vi "test Check If Custom Device is Enabled.vi"(8 "error in":errorcluster, 11 "TestCase in":refnum<class "Scripting.lvclass">) -> (0 "error out":errorcluster)   [LabVIEW 2020, in "Scripting.lvclass"]
uses:
  Scripting.lvclass
  Scripting/Ballard/Ballard ARINC 429 Scripting.lvlib
  <vilib>/addons/_JKI Toolkits/VI Tester/TestCase.llb/TestCase.lvclass
  C:/Program Files (x86)/National Instruments/LabVIEW 2020/vi.lib/addons/_JKI Toolkits/VI Tester/TestCase.llb/TestCase.lvclass
  C:/dev/git/niveristand-ballard-arinc429-custom-device/Source/Custom Device Support/Tests/Unit/Scripting/Scripting.lvclass
panel:
  out "TestCase out":refnum<class "Scripting.lvclass">
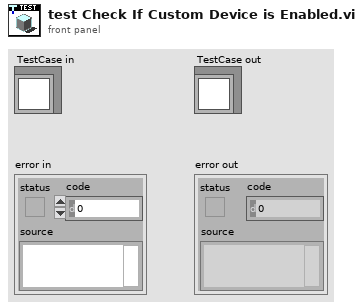
[diagram p1: front panel]
types:
  T1 = typedef "Custom Device API.lvlib/Custom Device Item Ref.ctl" = u64
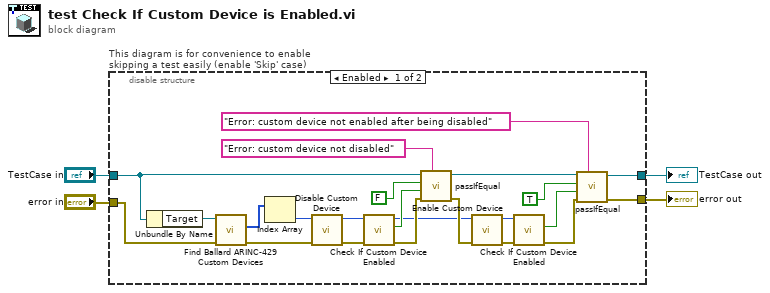
[diagram p0: block diagram]
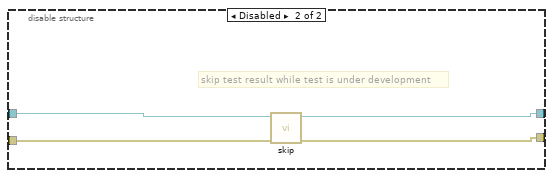
[diagram p2: hidden frame]
diagram:
  n1 = disable-structure "This diagram is for convenience to enable skipping a test easily (enable 'Skip' case)" shown="Enabled" {
    disable-tunnel: "TestCase in" -> [w20 w31]
    disable-tunnel: [w6 w29] -> w1
    disable-tunnel: [w7 w30] -> w3
    disable-tunnel: "error in" -> [w27 w28]
    frame Enabled {
      n2 = Unbundle By Name(w20) -> ("Target"=w22:refnum<k24>)
      n3 = call "Find Ballard ARINC-429 Custom Devices.vi"("error in"=w27, "target in"=w22) -> ("error out"=w23:errorcluster, "Ballard ARINC 429 custom devices"=w25:u64[])  [unwired: 7 in, 1 out]
      n4 = Index Array(array=w25) -> (element=w24:u64)  [unwired: 1 in]
      n5 = call "Disable Custom Device.vi"("error in (no error)"=w23, "Ballard ARINC 429 ref"=w24) -> ("error out"=w19:errorcluster, "Ballard ARINC 429 ref out"=w18:T1)  [unwired: 8 in]
      n6 = call "Check If Custom Device Enabled.vi"("error in (no error)"=w19, "Ballard ARINC 429 ref"=w18) -> ("error out"=w15:errorcluster, "Is Custom Device Enabled?"=w17:bool, "Ballard ARINC 429 ref"=w14:T1)  [unwired: 7 in]
      n7 = call-dynamic "passIfEqual.vi"("custom report message (\"\")"="Error: custom device not disabled" ("custom report message (\"\")"), "error in (no error)"=w15, "y"=w17, "x"=FALSE, "TestCase in"=w20) -> ("error out"=w26:errorcluster, "TestCase out"=w5:refnum<class "Scripting.lvclass">)  [unwired: 5 in]
      n8 = call "Enable Custom Device.vi"("error in (no error)"=w26, "Ballard ARINC 429 ref"=w14) -> ("error out"=w11:errorcluster, "Ballard ARINC 429 ref out"=w10:T1)  [unwired: 8 in]
      n9 = call "Check If Custom Device Enabled.vi"("error in (no error)"=w11, "Ballard ARINC 429 ref"=w10) -> ("error out"=w9:errorcluster, "Is Custom Device Enabled?"=w8:bool)  [unwired: 7 in, 1 out]
      n10 = call-dynamic "passIfEqual.vi"("custom report message (\"\")"="Error: custom device not enabled after being disabled" ("custom report message (\"\")"), "error in (no error)"=w9, "y"=w8, "x"=TRUE, "TestCase in"=w5) -> ("error out"=w7:errorcluster, "TestCase out"=w6:refnum<class "Scripting.lvclass">)  [unwired: 5 in]
    }
    frame Disabled {
      # "skip test result while test is under development"
      n11 = call <vilib>:"skip.vi"("error in (no error)"=w28, "TestCase in"=w31) -> ("error out"=w30:errorcluster, "TestCase out"=w29:refnum<class "Scripting.lvclass">)  [unwired: 8 in]
    }
  }
  "error out" <- w3
  "TestCase out" <- w1
